vi "autonDistance.vi"(0 "RobotDriveDevRef":T3={"DevStatus"={"status"=FALSE, "code"=0, "source"=""}, "Motors[]"=[], "Square Inputs"=FALSE, "Max Output"=1.0}, 5 "navX Device":T1={"Interface"={"Protocol"=enum."SERIAL", "Update Rate (4Hz-60Hz)"=4, "navX Open TypeDef"=variant}, "Notify Packet"=refnum, "Loop VI Refnum"=refnum, "Ready to Close Occurrence Refnum"=refnum} {"Interface"."Update Rate (4Hz-60Hz)" min=4 max=60 step=1}, 9 "Reset":bool, 11 "Numeric":dbl) -> (4 "s? t:f":bool, 6 "RobotDriveDevRef 2":T3={"DevStatus"={"status"=FALSE, "code"=0, "source"=""}, "Motors[]"=[], "Square Inputs"=FALSE, "Max Output"=1.0}, 8 "Yaw 2":cluster{"t":dbl, "Yaw":dbl}(graph), 10 "Waveform Chart":T11(graph), 15 "navX Device 2":T1={"Interface"={"Protocol"=enum."SERIAL", "Update Rate (4Hz-60Hz)"=4, "navX Open TypeDef"=variant}, "Notify Packet"=refnum, "Loop VI Refnum"=refnum, "Ready to Close Occurrence Refnum"=refnum} {"Interface"."Update Rate (4Hz-60Hz)" min=4 max=60 step=1})   [LabVIEW 2015]
uses:
  <vilib>/Rock Robotics/WPI/RobotDrive/WPI_RobotDriveDevRef.ctl
  <vilib>/Rock Robotics/WPI/MotorControl/WPI_MotorControlDeviceRef.ctl
  <vilib>/Rock Robotics/WPI/MotorControl/WPI_MotorControlType.ctl
  <vilib>/Rock Robotics/SystemInterfaces/DIO/FPGA_DIOPWMChannel.ctl
  <vilib>/Rock Robotics/WPI/PWM/WPI_PWMDeadband.ctl
  <vilib>/Rock Robotics/WPI/CAN/Jaguar/SubVIs/WPI_CANJaguar_ControlMode.ctl
  <vilib>/Rock Robotics/WPI/CAN/TalonSRX/WPI_CANTalonSRX_APIControlMode.ctl
  navX-MXP-LabVIEW/navX Library v2/TypeDefs/Z900_navX_DeviceTypeDef.ctl
  navX-MXP-LabVIEW/navX Library v2/TypeDefs/Z900_navX_ProtocolTypeDef.ctl
  navX-MXP-LabVIEW/navX Library v2/TypeDefs/Z900_navX_NotifyPacketTypeDef.ctl
  navX-MXP-LabVIEW/navX Library v2/TypeDefs/Z900_navX_ActionTypeDef.ctl
  <vilib>/addons/control/pid/pid.llb/PID (DBL).vi
  <vilib>/addons/control/pid/NI_PID_pid.lvlib
  navX-MXP-LabVIEW/navX Library v2/navX Library v2.lvlib
panel:
  in  "index 2":i32
  in  "index":i32
  out "PID output":dbl
  out "Yaw":dbl
  out "Fused Heading":dbl(knob) scale=0.0..360.0
  out "Sensor Position 2":dbl
  out "Sensor Position":dbl
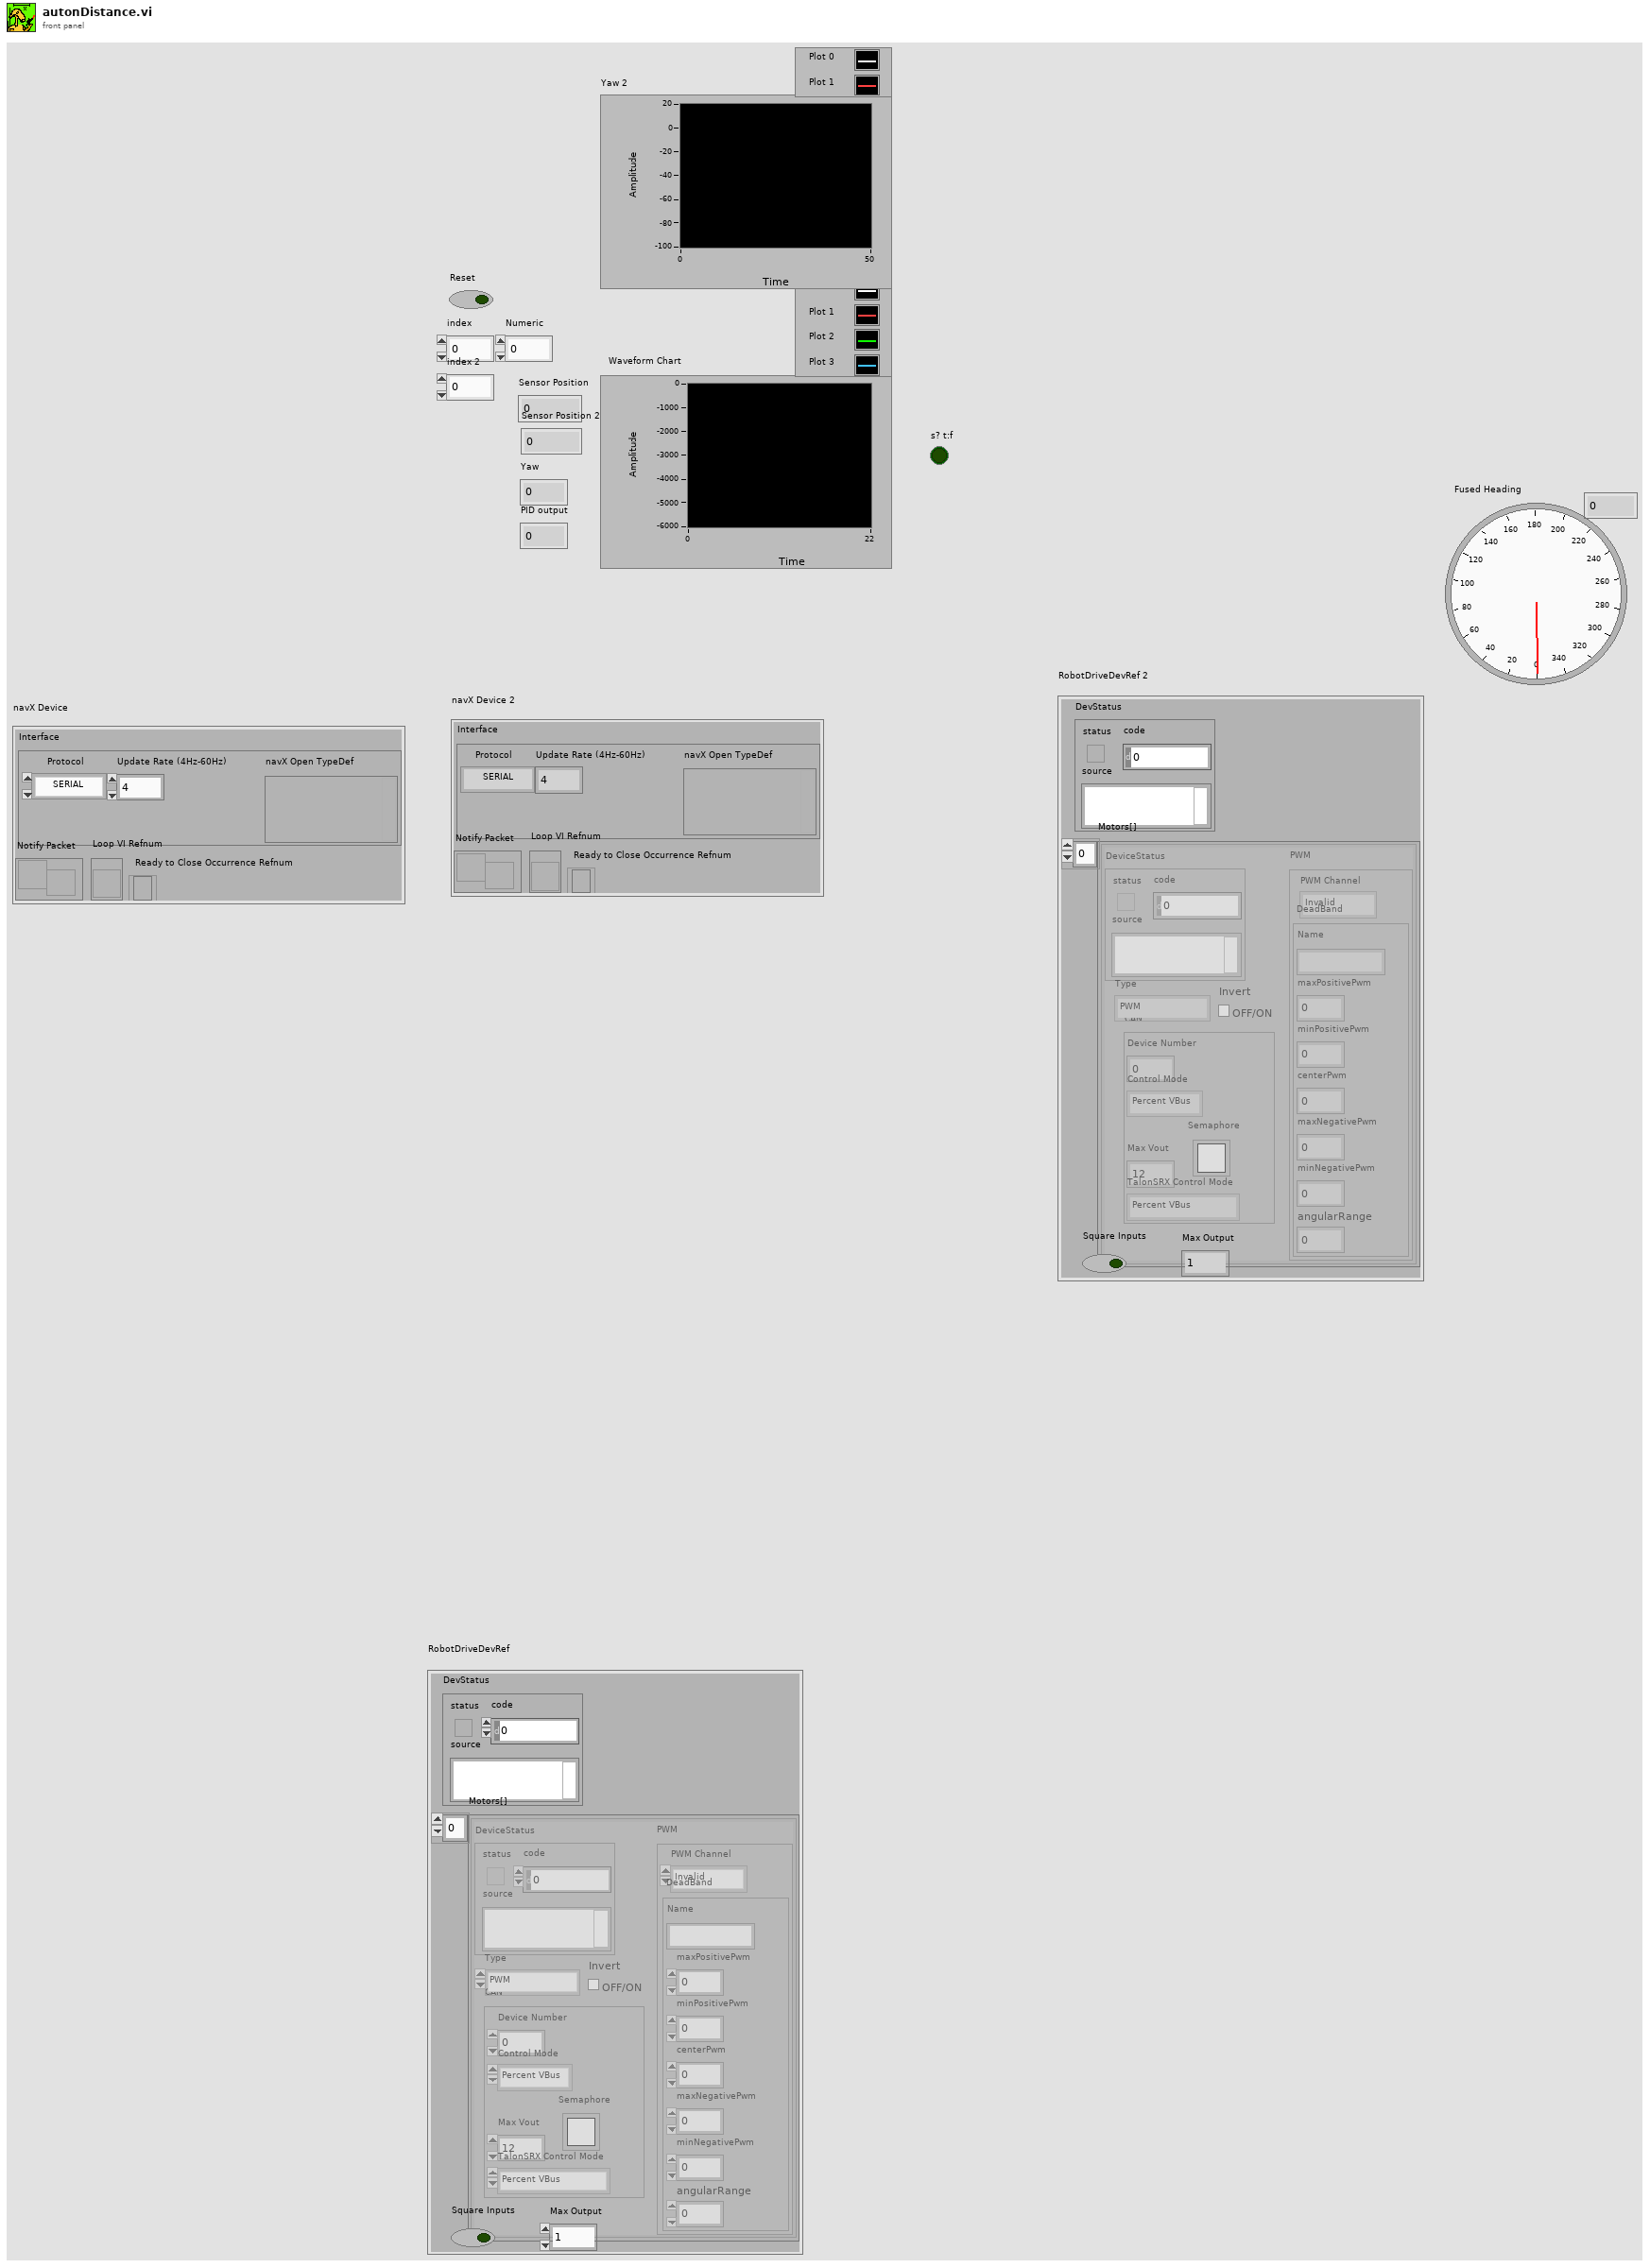
[diagram p1: front panel]
types:
  T1 = typedef "navX Library v2.lvlib/Z900_navX_DeviceTypeDef.ctl" = cluster{"Interface":cluster{"Protocol":T2, "Update Rate (4Hz-60Hz)":u8, "navX Open TypeDef":variant}, "Notify Packet":refnum<notifier>, "Loop VI Refnum":refnum<vi>, "Ready to Close Occurrence Refnum":refnum<k4>}
  T2 = typedef "navX Library v2.lvlib/Z900_navX_ProtocolTypeDef.ctl" = enum16{"SERIAL", "I2C", "SPI"}
  T3 = typedef "WPI_RobotDriveDevRef.ctl" = cluster{"DevStatus":errorcluster, "Motors[]":T4[], "Square Inputs":bool, "Max Output":dbl}
  T4 = typedef "WPI_MotorControlDeviceRef.ctl" = cluster{"DeviceStatus":errorcluster, "Type":T5, "PWM":cluster{"PWM Channel":T6, "DeadBand":T7}, "CAN":cluster{"Device Number":u8, "Control Mode":T8, "Semaphore":T9, "Max Vout":dbl, "TalonSRX Control Mode":T10}, "Invert":bool}
  T5 = typedef "WPI_MotorControlType.ctl" = enum16{"PWM", "CAN", "CANTalonSRX"}
  T6 = typedef "FPGA_DIOPWMChannel.ctl" = enum8{"PWM 0", "PWM 1", "PWM 2", "PWM 3", "PWM 4", "PWM 5", "PWM 6", "PWM 7", "PWM 8", "PWM 9", "PWM MXP 0", "PWM MXP 1", "PWM MXP 2", "PWM MXP 3", "PWM MXP 4", "PWM MXP 5", "PWM MXP 6", "PWM MXP 7", "PWM MXP 8", "PWM MXP 9", "Invalid"}
  T7 = typedef "WPI_PWMDeadband.ctl" = cluster{"Name":string, "maxPositivePwm":i32, "minPositivePwm":i32, "centerPwm":i32, "maxNegativePwm":i32, "minNegativePwm":i32, "angularRange":u16}
  T8 = typedef "WPI_CANJaguar_ControlMode.ctl" = enum8{"Percent VBus", "Current", "Speed", "Position", "Voltage"}
  T9 = typedef "Semaphore RefNum" = refnum<k1>
  T10 = typedef "WPI_CANTalonSRX_APIControlMode.ctl" = enum8{"Percent VBus", "Speed", "Position", "Slave", "Unchanged / Invalid", "Voltage Compensation", "Current", "Motion Profile"}
  T11 = cluster{"Encoder Position":dbl, "Encoder Index Count":dbl, "Encoder Position":dbl, "Encoder Index Count":dbl}
  T12 = cluster{"proportional gain (Kc)":dbl, "integral time (Ti, min)":dbl, "derivative time (Td, min)":dbl}
  T13 = cluster{"Yaw":dbl, "Roll":dbl, "Pitch":dbl, "Heading":dbl, "Fused Heading":dbl}
  T14 = typedef "WPI_CANTalonSRX_GlobalStatus.ctl" = cluster{"Applied Throttle":dbl, "Module Enabled":bool, "CAN Error":errorcluster, "Closed Loop Error":dbl, "Forward Limit Switch Closed":bool, "Reverse Limit Switch Closed":bool, "Sensor Position":dbl, "Sensor Velocity":dbl, "Current":dbl, "Sticky Fault - Over Temp":bool, "Sticky Fault - Under Voltage":bool, "Sticky Fault - Forward Limit":bool, "Sticky Fault - Reverse Limit":bool, "Sticky Fault - Forward Soft Limit":bool, "Sticky Fault - Reverse Soft Limit":bool, "Brake is Enabled":bool, "Encoder Position":dbl, "Encoder Velocity":dbl, "Encoder Index Count":dbl, "Encoder A Pin State":bool, "Encoder B Pin State":bool, "Encoder Index Pin State":bool, "Analog In":dbl, "Analog In Velocity":dbl, "Temperature (C)":dbl, "Battery Voltage":dbl, "Control 5 Is Supported":bool, "Current Profile Slot Select":dbl, "Pos Div 8":bool, "Vel Div 4":bool, "Pulse Width Position":i32, "Pulse Width Velocity":i32, "Pulse Width Rise To Rise (us)":i32, "Pulse Width Rise To Fall (us)":i32, "Mot Prof Active Is Under Run":bool, "Mot Prof Active Has Under Run":bool, "Mot Prof Active Is Last":bool, "Mot Prof Active Velocity Only":bool, "Mot Prof Active Is Valid":bool, "Mot Prof Buffer Is Full":bool, "Mot Prof Active Profile Slot Select":i32, "Mot Prof NextID":i32, "Mot Prof Count":i32, "Mot Prof Active Velocity":dbl, "Mot Prof Active Position":dbl, "Mot Prof Output Enable":i32}
  T15 = cluster{dbl, "Encoder Index Count":dbl, "Encoder Position":dbl, "Encoder Index Count":dbl}
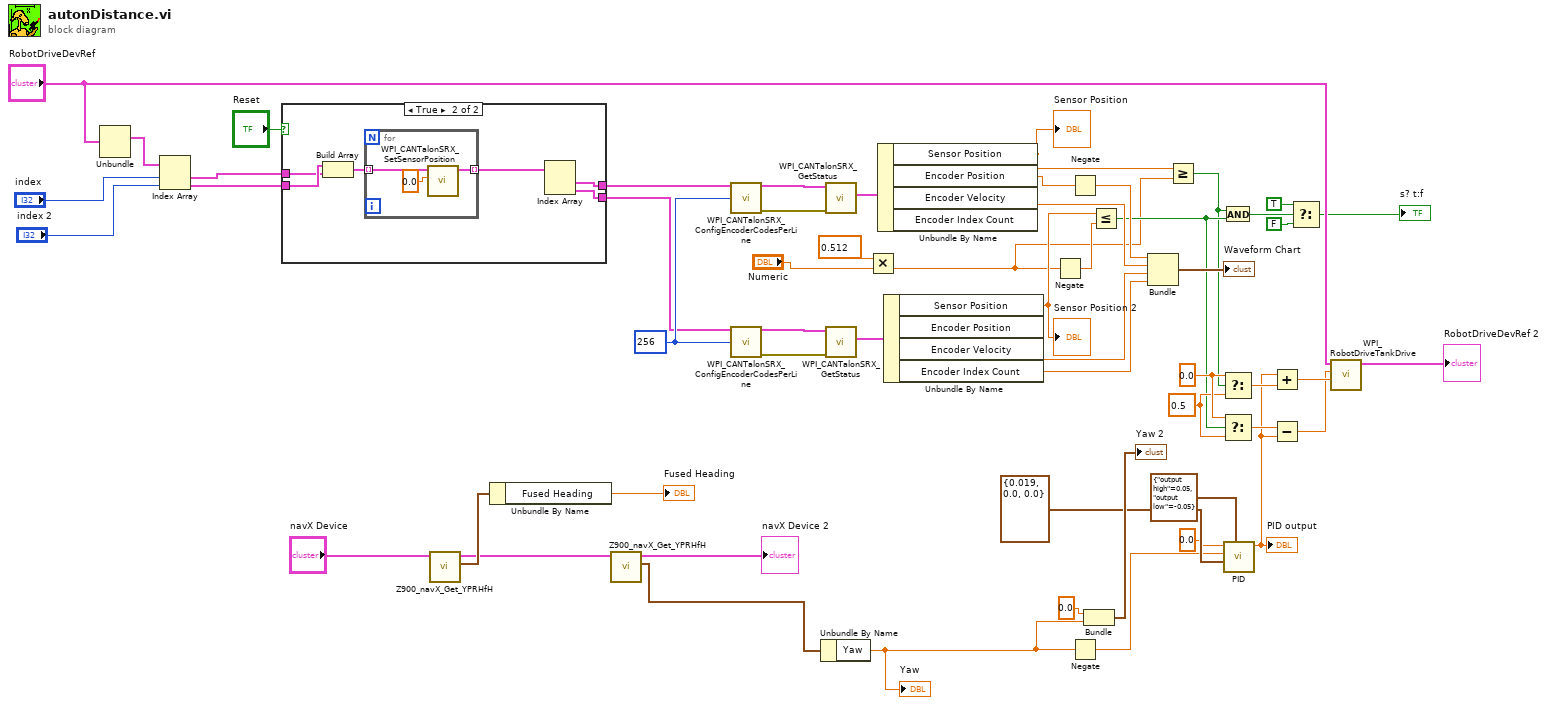
[diagram p0: block diagram]
diagram:
  w33 = 0.5 ("f")
  w36 = 0.0 ("t")
  w45 = u32 256 ("Number Encoder Lines\n(Counts Per Rotation)")
  n1 = Unbundle("RobotDriveDevRef") -> ("Motors[]"=w17:T4[])  [unwired: 3 out]
  n2 = Index Array(array=w17, index #1="index", index #2="index 2") -> (element #1=w16:T4, element #2=w15:T4)
  n3 = case shown="True" "Reset" {
    tunnel: w15 -> [w57 w63]
    tunnel: w16 -> [w56 w62]
    tunnel: [w57 w59] -> w43
    tunnel: [w56 w58] -> w42
    frame False {
    }
    frame True {
      n4 = Build Array(w63, w62) -> (w61:T4[])
      n5 = for {
        tunnel: w61 -> [w66] mode=indexing
        tunnel: [w64] -> w60 mode=indexing
        n6 = call <vilib>:"WPI_CANTalonSRX_SetSensorPosition.vi"("New Sensor Position"=0.0, "CAN Talon SRX Ref"=w66) -> ("CAN Talon SRX Ref"=w64:T4)  [unwired: 8 in, 1 out]
      }
      n7 = Index Array(array=w60) -> (element #1=w59:T4, element #2=w58:T4)  [unwired: 2 in]
    }
  }
  n8 = call "Z900_navX_Get_YPRHfH.vi"("navX Device"="navX Device") -> ("YRPHfH"=w6:T13, "navX Device"=w2:T1)  [unwired: 7 in, 2 out]
  n9 = Unbundle By Name(w6) -> ("Fused Heading"=→"Fused Heading":dbl)
  n10 = call "Z900_navX_Get_YPRHfH.vi"("navX Device"=w2) -> ("YRPHfH"=w3:T13, "navX Device"=→"navX Device 2":T1)  [unwired: 7 in, 2 out]
  n11 = call <vilib>:"WPI_CANTalonSRX_ConfigEncoderCodesPerLine.vi"("CAN Talon SRX Ref"=w43, "Number Encoder Lines\n(Counts Per Rotation)"=w45) -> ("CAN Talon SRX Ref"=w48:T4, "error out"=w49:errorcluster)  [unwired: 12 in]
  n12 = call <vilib>:"WPI_CANTalonSRX_ConfigEncoderCodesPerLine.vi"("CAN Talon SRX Ref"=w42, "Number Encoder Lines\n(Counts Per Rotation)"=w45) -> ("CAN Talon SRX Ref"=w46:T4, "error out"=w47:errorcluster)  [unwired: 12 in]
  n13 = Unbundle By Name(w3) -> ("Yaw"=w25:dbl)
  "Yaw" <- w25
  n14 = call <vilib>:"WPI_CANTalonSRX_GetStatus.vi"("error in (no error)"=w49, "CAN Talon SRX Ref"=w48) -> ("Talon SRX Status"=w54:T14)  [unwired: 7 in, 2 out]
  n15 = call <vilib>:"WPI_CANTalonSRX_GetStatus.vi"("error in (no error)"=w47, "CAN Talon SRX Ref"=w46) -> ("Talon SRX Status"=w55:T14)  [unwired: 7 in, 2 out]
  n16 = Multiply(x=0.512, y="Numeric") -> (x*y=w10:dbl)
  n17 = Unbundle By Name(w54) -> ("Sensor Position"=w35:dbl, "Encoder Position"=w53:dbl, "Encoder Index Count"=w52:dbl)  [unwired: 1 out]
  "Sensor Position" <- w35
  n18 = Unbundle By Name(w55) -> ("Sensor Position"=w34:dbl, "Encoder Position"=w51:dbl, "Encoder Index Count"=w50:dbl)  [unwired: 1 out]
  "Sensor Position 2" <- w34
  n19 = Negate(x=w10) -> (-x=w12:dbl)
  n20 = Negate(x=w53) -> (-x=w40:dbl)
  n21 = Negate(x=w25) -> (-x=w19:dbl)
  n22 = Bundle("t"=0.0, "Yaw"=w25) -> (→"Yaw 2":cluster{"t":dbl, "Yaw":dbl})  [unwired: 1 in]
  n23 = Less Or Equal?(x=w34, y=w12) -> (x <= y?=w32:bool)
  n24 = Bundle(w40, "Encoder Index Count"=w52, "Encoder Position"=w51, "Encoder Index Count"=w50) -> (→"Waveform Chart":T15)  [unwired: 1 in]
  n25 = Greater Or Equal?(x=w35, y=w10) -> (x >= y?=w31:bool)
  n26 = And(x=w31, y=w32) -> (x .and. y?=w39:bool)
  n27 = Select(t=w36, s=w31, f=w33) -> (s? t:f=w30:dbl)
  n28 = Select(t=w36, s=w32, f=w33) -> (s? t:f=w29:dbl)
  n29 = call-poly <vilib>:"PID.vi"("output range"=cluster{"output high":dbl, "output low":dbl} {"output high"=0.05, "output low"=-0.05}, "PID gains"=T12 {"proportional gain (Kc)"=0.019, "integral time (Ti, min)"=0.0, "derivative time (Td, min)"=0.0}, "process variable"=w19, "setpoint"=0.0 ("t")) -> ("output"=w20:dbl)  [unwired: 6 in, 1 out]
  "PID output" <- w20
  n30 = Add(x=w20, y=w30) -> (x+y=w22:dbl)
  n31 = Subtract(x=w29, y=w20) -> (x-y=w21:dbl)
  n32 = Select(t=TRUE, s=w39, f=FALSE) -> (s? t:f=→"s? t:f":bool)
  n33 = call <vilib>:"WPI_RobotDriveTankDrive.vi"("Right axis value"=w22, "Left axis value"=w21, "RobotDriveDevRef"="RobotDriveDevRef") -> ("RobotDriveDevRef"=→"RobotDriveDevRef 2":T3)  [unwired: 6 in, 2 out]
